vi "SMU2 Trigger Pulse.vi"() -> ()   [LabVIEW 2010]
uses:
  <instrlib>/Keithley 24XX/Keithley 24XX.lvlib
panel:
  out "error out":errorcluster
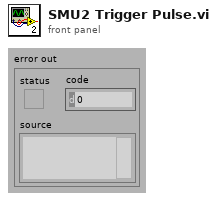
[diagram p1: front panel]
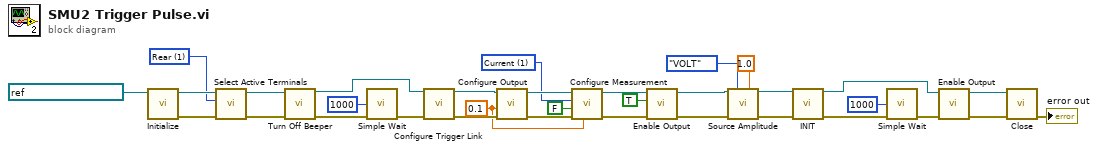
[diagram p0: block diagram]
diagram:
  w10 = u16 1 items=["Volts", "Current", "Resistance"] ("Function (0: Volts)")
  w9 = 0.1 ("Compliance  Level (0.1)")
  w11 = u16 1 items=["Front", "Rear"] ("Active Terminals (0: Front)")
  n1 = call <instrlib>:"Initialize.vi"("VISA resource name"=refnum<visa-resource-name> "GPIB0::10::INSTR") -> ("error out"=w33:errorcluster, "VISA resource name out"=w22:refnum<visa-resource-name>)  [unwired: 9 in]
  n2 = call <instrlib>:"Select Active Terminals.vi"("error in (no error)"=w33, "Active Terminals (0: Front)"=w11, "VISA resource name"=w22) -> ("error out"=w32:errorcluster, "VISA resource name out"=w21:refnum<visa-resource-name>)  [unwired: 7 in]
  n3 = call "Turn Off Beeper.vi"("VISA resource name"=w21, "error in (no error)"=w32) -> ("VISA resource name out"=w20:refnum<visa-resource-name>, "error out"=w31:errorcluster)  [unwired: 12 in]
  n4 = call "Simple Wait.vi"("mS"=u32 1000, "error in"=w31) -> ("error out"=w29:errorcluster)  [unwired: 12 in, 1 out]
  n5 = call <instrlib>:"Configure Trigger Link.vi"("VISA resource name"=w20, "error in (no error)"=w29) -> ("VISA resource name out"=w19:refnum<visa-resource-name>, "error out"=w28:errorcluster)  [unwired: 12 in]
  n6 = call <instrlib>:"Configure Output.vi"("error in (no error)"=w28, "Compliance  Level (0.1)"=w9, "VISA resource name"=w19) -> ("error out"=w27:errorcluster, "VISA resource name out"=w18:refnum<visa-resource-name>)  [unwired: 7 in]
  n7 = call <instrlib>:"Configure Measurement.vi"("Manual Range (1.0)"=w9, "error in (no error)"=w27, "Enable Auto Range (T:Enable)"=FALSE, "Function (0: Volts)"=w10, "VISA resource name"=w18) -> ("error out"=w26:errorcluster, "VISA resource name out"=w17:refnum<visa-resource-name>)  [unwired: 5 in]
  n8 = call <instrlib>:"Enable Output.vi"("error in (no error)"=w26, "Enable Output (T: Enable)"=TRUE, "VISA resource name"=w17) -> ("error out"=w25:errorcluster, "VISA resource name out"=w16:refnum<visa-resource-name>)  [unwired: 7 in]
  n9 = call "Source Amplitude.vi"("VISA resource name"=w16, "Source Function"=enum16{"CURR", "VOLT"}."VOLT", "Source Level"=1.0, "error in (no error)"=w25) -> ("VISA resource name out"=w15:refnum<visa-resource-name>, "error out"=w24:errorcluster)  [unwired: 10 in]
  n10 = call "INIT.vi"("VISA resource name"=w15, "error in (no error)"=w24) -> ("VISA resource name out"=w3:refnum<visa-resource-name>, "error out"=w2:errorcluster)  [unwired: 12 in]
  n11 = call "Simple Wait.vi"("mS"=u32 1000, "error in"=w2) -> ("error out"=w1:errorcluster)  [unwired: 12 in, 1 out]
  n12 = call <instrlib>:"Enable Output.vi"("error in (no error)"=w1, "VISA resource name"=w3) -> ("error out"=w23:errorcluster, "VISA resource name out"=w14:refnum<visa-resource-name>)  [unwired: 8 in]
  n13 = call <instrlib>:"Close.vi"("error in (no error)"=w23, "VISA resource name"=w14) -> ("error out"=→"error out":errorcluster)  [unwired: 9 in]
